vi "test_Measurement_Measure_StreamsExpectedResults.vi"(8 "error in":errorcluster) -> (0 "error out":errorcluster, 2 "result":string, 3 "pass":bool)   [LabVIEW 2021, in "MeasurementServerTests.lvlib" / "Measurement Service Tests.lvlib"]
uses:
  Measurement Service Tests.lvlib
  Continuous Counting Measurement2/Run Service.vi
  Continuous Counting Measurement/Run Non-reentrant Service.vi
  Continuous Counting Measurement2/Continuous Counting Measurement2.lvclass
  Continuous Counting Measurement/Continuous Counting Measurement.lvclass
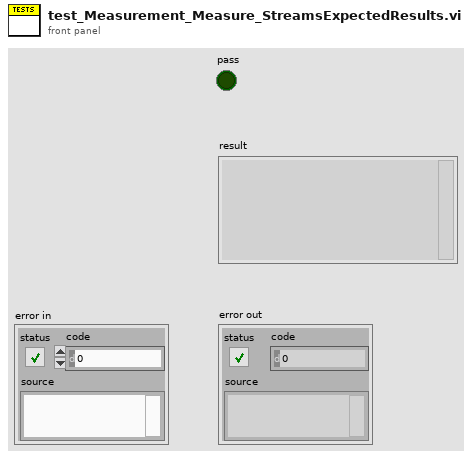
[diagram p1: front panel]
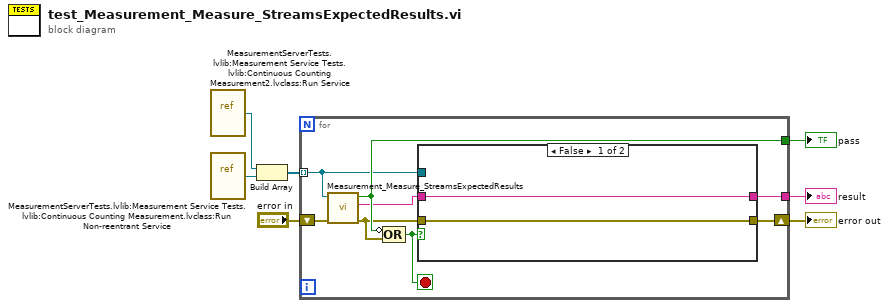
[diagram p0: block diagram]
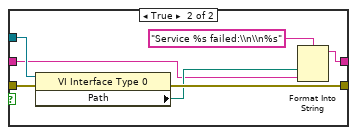
[diagram p2: hidden frame]
diagram:
  n1 = vi-ref "MeasurementServerTests.lvlib:Measurement Service Tests.lvlib:Continuous Counting Measurement2.lvclass:Run Service.vi"() -> (w3:refnum<vi>)
  n2 = vi-ref "MeasurementServerTests.lvlib:Measurement Service Tests.lvlib:Continuous Counting Measurement.lvclass:Run Non-reentrant Service.vi"() -> (w2:refnum<vi>)
  n3 = Build Array(w3, w2) -> (w1:refnum<vi>[])
  n4 = for {
    tunnel: [w11] -> w5
    tunnel: [w14] -> w4
    shift-right: [w8] -> w6
    shift-left: "error in" -> [w15]
    tunnel: w1 -> [w10] mode=indexing
    stop <- w13 stop-if-true
    n5 = call "Measurement_Measure_StreamsExpectedResults.vi"("error in"=w15, "run service vi"=w10) -> ("error out"=w9:errorcluster, "result"=w12:string, "pass"=w14:bool)  [unwired: 7 in]
    n6 = Compound Arithmetic op=OR(invert w14, w9) -> (w13:bool)
    n7 = case shown="False" w13 {
      tunnel: w12 -> [w17 w19]
      tunnel: [w17 w18] -> w11
      tunnel: w10 -> [_ w24]
      tunnel: w9 -> [w16 w23]
      tunnel: [w16 w22] -> w8
      frame False {
      }
      frame True {
        n8 = property class="VI Interface Type 0"(reference=w24, error in=w23) -> (error out=w22:errorcluster, "Path"=w20:path)  [unwired: 1 out]
        n9 = Format Into String(format string="Service %s failed:\\n\\n%s", w20, w19) -> (resulting string=w18:string)  [unwired: 2 in, 1 out]
      }
    }
  }
  "pass" <- w4
  "result" <- w5
  "error out" <- w6
